vi "Asynch Timer Loop.vi"(8 "error in (no error)":errorcluster, 9 "Instance Name":string, 10 "Timer Setup Params Notifier":refnum<notifier>, 11 "Timer State Rtn event":refnum<user-event>) -> ()   [LabVIEW 2015, in "Tool Module.lvlib"]
uses:
  Tool Module.lvlib
  Timer Setup Params Typedef.ctl
  Timer State Return Typedef.ctl
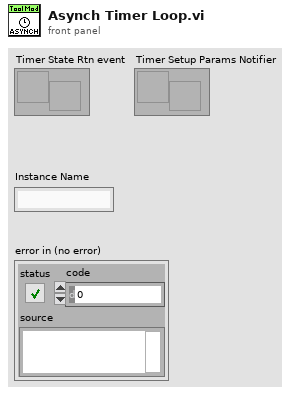
[diagram p1: front panel]
types:
  T1 = typedef "Tool Module.lvlib/Timer State Return Typedef.ctl" = cluster{"Instance Name":string, "On/Off":bool, "Running":bool}
  T2 = typedef "Tool Module.lvlib/Timer Setup Params Typedef.ctl" = cluster{"Timer On":bool, "Period":i32, "Count":i32}
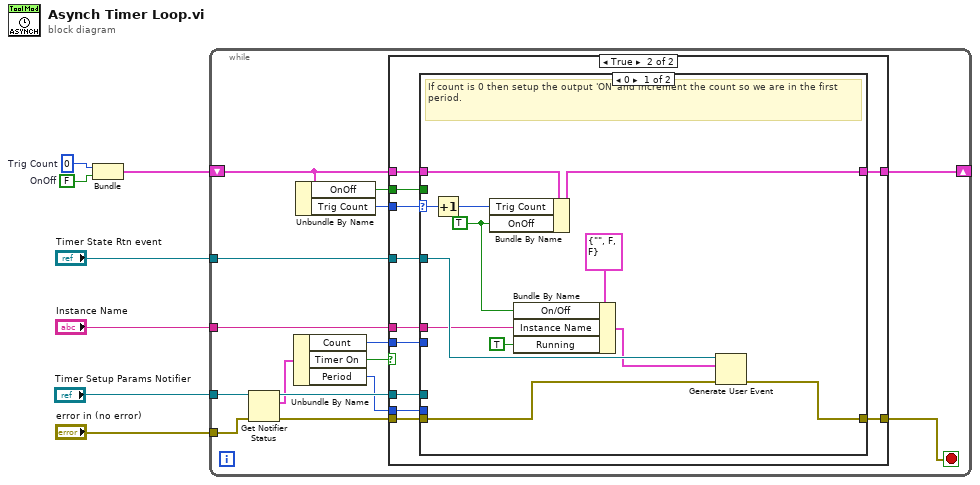
[diagram p0: block diagram]
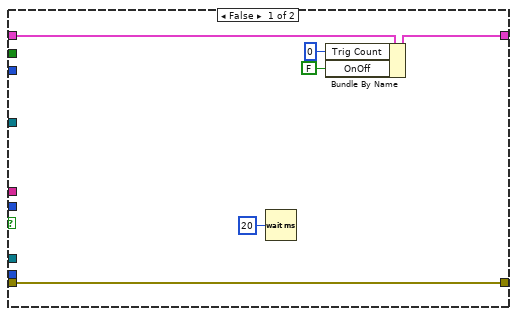
[diagram p2: hidden frame]
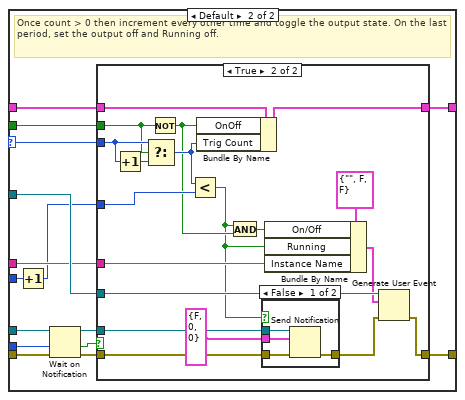
[diagram p3: hidden frame]
diagram:
  w3 = FALSE  # OnOff
  w4 = 0  # Trig Count
  n1 = Bundle("Trig Count"=w4, "OnOff"=w3) -> (w2:cluster{"Trig Count":i32, "OnOff":bool})  [unwired: 1 in]
  n2 = while {
    tunnel: "Timer State Rtn event" -> [w19]
    tunnel: "Instance Name" -> [w18]
    tunnel: "Timer Setup Params Notifier" -> [w17]
    tunnel: "error in (no error)" -> [w16]
    shift-right: [w10] -> _
    shift-left: w2 -> [w12]
    stop <- w20 stop-if-true
    n3 = Get Notifier Status(notifier=w17, error in (no error)=w16) -> (notifier out=w21:refnum<notifier>, current notification=w15:T2, error out=w22:errorcluster)  [unwired: 2 out]
    n4 = Unbundle By Name(w15) -> ("Count"=w8:i32, "Timer On"=w13:bool, "Period"=w14:i32)
    n5 = Unbundle By Name(w12) -> ("OnOff"=w9:bool, "Trig Count"=w11:i32)
    n6 = case shown="True" w13 {
      tunnel: w22 -> [w28 w39]
      tunnel: w21 -> [_ w38]
      tunnel: [w28 w37] -> w20
      tunnel: w19 -> [_ w36]
      tunnel: w18 -> [_ w35]
      tunnel: w14 -> [_ w34]
      tunnel: w12 -> [w26 w33]
      tunnel: w11 -> [_ w32]
      tunnel: [w25 w31] -> w10
      tunnel: w9 -> [_ w30]
      tunnel: w8 -> [_ w29]
      frame False {
        n7 = Wait (ms)(milliseconds to wait=u32 20) -> ()  [unwired: 1 out]
        n8 = Bundle By Name(cluster=w26, "Trig Count"=0, "OnOff"=FALSE) -> (w25:cluster{"Trig Count":i32, "OnOff":bool})
      }
      frame True {
        n9 = case shown="0" w32 {
          selector: w32 -> [w48 w54]
          tunnel: w39 -> [w46 w66]
          tunnel: w38 -> [_ w64]
          tunnel: [w51 w62] -> w37
          tunnel: w36 -> [w50 w61]
          tunnel: w35 -> [w43 w60]
          tunnel: w34 -> [_ w59]
          tunnel: w33 -> [w49 w58]
          tunnel: [w47 w57] -> w31
          tunnel: w30 -> [_ w56]
          tunnel: w29 -> [_ w53]
          frame 0 {
            w42 = TRUE ("OnOff")
            # "If count is 0 then setup the output 'ON' and increment the count so we are in the first period."
            n10 = Increment(x=w48) -> (x+1=w45:i32)
            n11 = Bundle By Name(cluster=w49, "Trig Count"=w45, "OnOff"=w42) -> (w47:cluster{"Trig Count":i32, "OnOff":bool})
            n12 = Bundle By Name(cluster=T1 {"Instance Name"="", "On/Off"=FALSE, "Running"=FALSE} ("_Trigger State Rtn Params Typedef"), "On/Off"=w42, "Instance Name"=w43, "Running"=TRUE) -> (w41:T1)
            n13 = Generate User Event(user event=w50, event data cluster=w41, error in=w46) -> (error out=w51:errorcluster)  [unwired: 1 in, 1 out]
          }
          frame Default {
            # "Once count > 0 then increment every other time and toggle the output state. On the last period, set the output off and Running off."
            n14 = Increment(x=w53) -> (x+1=w52:i32)
            n15 = Wait on Notification(notifier=w64, timeout in ms (-1)=w59, error in (no error)=w66) -> (notifier out=w55:refnum<notifier>, timed out?=w65:bool, error out=w63:errorcluster)  [unwired: 1 in, 1 out]
            n16 = case shown="True" w65 {
              tunnel: w63 -> [w68 w74]
              tunnel: [w68 w87] -> w62
              tunnel: w61 -> [_ w86]
              tunnel: w60 -> [_ w79]
              tunnel: w58 -> [w67 w85]
              tunnel: w54 -> [_ w83]
              tunnel: [w67 w69] -> w57
              tunnel: w56 -> [_ w82]
              tunnel: w55 -> [_ w72]
              tunnel: w52 -> [_ w77]
              frame False {
                # "This state shouldn't happen."
              }
              frame True {
                n17 = Increment(x=w83) -> (x+1=w84:i32)
                n18 = Select(t=w83, s=w82, f=w84) -> (s? t:f=w78:i32)
                n19 = Not(x=w82) -> (.not. x?=w76:bool)
                n20 = Less?(x=w78, y=w77) -> (x < y?=w70:bool)
                n21 = Bundle By Name(cluster=w85, "OnOff"=w76, "Trig Count"=w78) -> (w69:cluster{"Trig Count":i32, "OnOff":bool})
                n22 = And(x=w70, y=w76) -> (x .and. y?=w75:bool)
                n23 = case shown="False" w70 {
                  tunnel: w74 -> [w91 w92]
                  tunnel: [w90 w92] -> w73
                  tunnel: w72 -> [w89 _]
                  tunnel: T2 {"Timer On"=FALSE, "Period"=0, "Count"=0} ("_Trigger Params Typedef") -> [w88 _]
                  frame False {
                    n24 = Send Notification(notification=w88, notifier=w89, error in (no error)=w91) -> (error out=w90:errorcluster)  [unwired: 1 out]
                  }
                  frame True {
                  }
                }
                n25 = Bundle By Name(cluster=T1 {"Instance Name"="", "On/Off"=FALSE, "Running"=FALSE} ("_Trigger State Rtn Params Typedef"), "On/Off"=w75, "Running"=w70, "Instance Name"=w79) -> (w80:T1)
                n26 = Generate User Event(user event=w86, event data cluster=w80, error in=w73) -> (error out=w87:errorcluster)  [unwired: 1 in, 1 out]
              }
            }
          }
        }
      }
    }
  }
